vi "Connect PV.vi"(8 "error in (no error)":errorcluster, 10 "PV URL":string, 11 "CS++DSCMonitor in":refnum<class "CS++DSCMonitor.lvclass">) -> (0 "error out":errorcluster, 3 "CS++DSCMonitor out":refnum<class "CS++DSCMonitor.lvclass">)   [LabVIEW 2014, in "CS++DSCMonitor.lvlib" / "CS++DSCMonitor.lvclass"]
doc: "Open connection to process variable."
uses:
  CS++DSCMonitor.lvclass
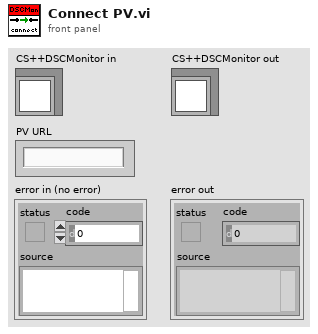
[diagram p1: front panel]
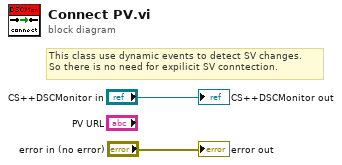
[diagram p0: block diagram]
diagram:
  # "This class use dynamic events to detect SV changes.\nSo there is no need for expilicit SV conntection."
  "error out" <- "error in (no error)"
  "CS++DSCMonitor out" <- "CS++DSCMonitor in"
